vi "Three part faster sub note on off.vi"() -> ()   [LabVIEW 2009]
uses:
  <vilib>/vision/Image Controls.llb/IMAQ Image.ctl
  <vilib>/Instr/_visa.llb/VISA Configure Serial Port (Instr).vi
  <vilib>/vision/NI_Vision_Development_Module.lvlib
panel:
  in  "Notes On/OFF":bool
  in  "VISA resource name":refnum<visa-resource-name>
  out "number":u8 format="%b"
  out "decimal integer string":string
  out "decimal integer string 2":string
  out "decimal integer string 3":string
  out "number 2":u8 format="%b"
  out "number 3":u8 format="%b"
  out "Guitar Cluster":T1
  out "Bass Cluster":T2
  out "Drum Cluster":T3
  out "Image 2":T4(plugin-control)
  in  "Orange Bass":T5={"Global Rectangle"=[220, 302, 227, 392], "Contours"=[{"ID"=enum."External", "Type"=2, "Coordinates"=[226, 391, 220, 302]}]} {"Contours"."Type" items=["No Selection", "Point", "Line", "Rectangle", "Oval", "Polygon", "Freehand Region", "Annulus", "Unused2", "Unused3", "Broken Line", "Freehand Line", "Rotated Rectangle"]}
  in  "Blue Bass":T5={"Global Rectangle"=[192, 292, 199, 386], "Contours"=[{"ID"=enum."External", "Type"=2, "Coordinates"=[192, 385, 198, 292]}]} {"Contours"."Type" items=["No Selection", "Point", "Line", "Rectangle", "Oval", "Polygon", "Freehand Region", "Annulus", "Unused2", "Unused3", "Broken Line", "Freehand Line", "Rotated Rectangle"]}
  in  "playtime":dbl=30.0
  in  "Orange Guitar":T5={"Global Rectangle"=[587, 282, 628, 378], "Contours"=[{"ID"=enum."External", "Type"=2, "Coordinates"=[627, 377, 587, 282]}]} {"Contours"."Type" items=["No Selection", "Point", "Line", "Rectangle", "Oval", "Polygon", "Freehand Region", "Annulus", "Unused2", "Unused3", "Broken Line", "Freehand Line", "Rotated Rectangle"]}
  in  "Yellow Guitar":T5={"Global Rectangle"=[546, 282, 563, 376], "Contours"=[{"ID"=enum."External", "Type"=2, "Coordinates"=[562, 375, 546, 282]}]} {"Contours"."Type" items=["No Selection", "Point", "Line", "Rectangle", "Oval", "Polygon", "Freehand Region", "Annulus", "Unused2", "Unused3", "Broken Line", "Freehand Line", "Rotated Rectangle"]}
  in  "Green Guitar":T5={"Global Rectangle"=[498, 284, 505, 376], "Contours"=[{"ID"=enum."External", "Type"=2, "Coordinates"=[498, 375, 504, 284]}]} {"Contours"."Type" items=["No Selection", "Point", "Line", "Rectangle", "Oval", "Polygon", "Freehand Region", "Annulus", "Unused2", "Unused3", "Broken Line", "Freehand Line", "Rotated Rectangle"]}
  in  "Blue Guitar":T5={"Global Rectangle"=[569, 290, 594, 372], "Contours"=[{"ID"=enum."External", "Type"=2, "Coordinates"=[593, 371, 569, 290]}]} {"Contours"."Type" items=["No Selection", "Point", "Line", "Rectangle", "Oval", "Polygon", "Freehand Region", "Annulus", "Unused2", "Unused3", "Broken Line", "Freehand Line", "Rotated Rectangle"]}
  in  "Red Guitar":T5={"Global Rectangle"=[526, 284, 530, 370], "Contours"=[{"ID"=enum."External", "Type"=2, "Coordinates"=[529, 369, 526, 284]}]} {"Contours"."Type" items=["No Selection", "Point", "Line", "Rectangle", "Oval", "Polygon", "Freehand Region", "Annulus", "Unused2", "Unused3", "Broken Line", "Freehand Line", "Rotated Rectangle"]}
  in  "Green Bass":T5={"Global Rectangle"=[100, 292, 131, 371], "Contours"=[{"ID"=enum."External", "Type"=2, "Coordinates"=[100, 370, 130, 292]}]} {"Contours"."Type" items=["No Selection", "Point", "Line", "Rectangle", "Oval", "Polygon", "Freehand Region", "Annulus", "Unused2", "Unused3", "Broken Line", "Freehand Line", "Rotated Rectangle"]}
  in  "Red Bass":T5={"Global Rectangle"=[129, 294, 154, 376], "Contours"=[{"ID"=enum."External", "Type"=2, "Coordinates"=[129, 375, 153, 294]}]} {"Contours"."Type" items=["No Selection", "Point", "Line", "Rectangle", "Oval", "Polygon", "Freehand Region", "Annulus", "Unused2", "Unused3", "Broken Line", "Freehand Line", "Rotated Rectangle"]}
  in  "Yellow Bass":T5={"Global Rectangle"=[160, 295, 175, 378], "Contours"=[{"ID"=enum."External", "Type"=2, "Coordinates"=[160, 377, 174, 295]}]} {"Contours"."Type" items=["No Selection", "Point", "Line", "Rectangle", "Oval", "Polygon", "Freehand Region", "Annulus", "Unused2", "Unused3", "Broken Line", "Freehand Line", "Rotated Rectangle"]}
  out "Image Dst Out":T4
  out "Frame Number":i32
  in  "Frame Start":i32
  in  "stop":bool
  in  "AVI Path":path
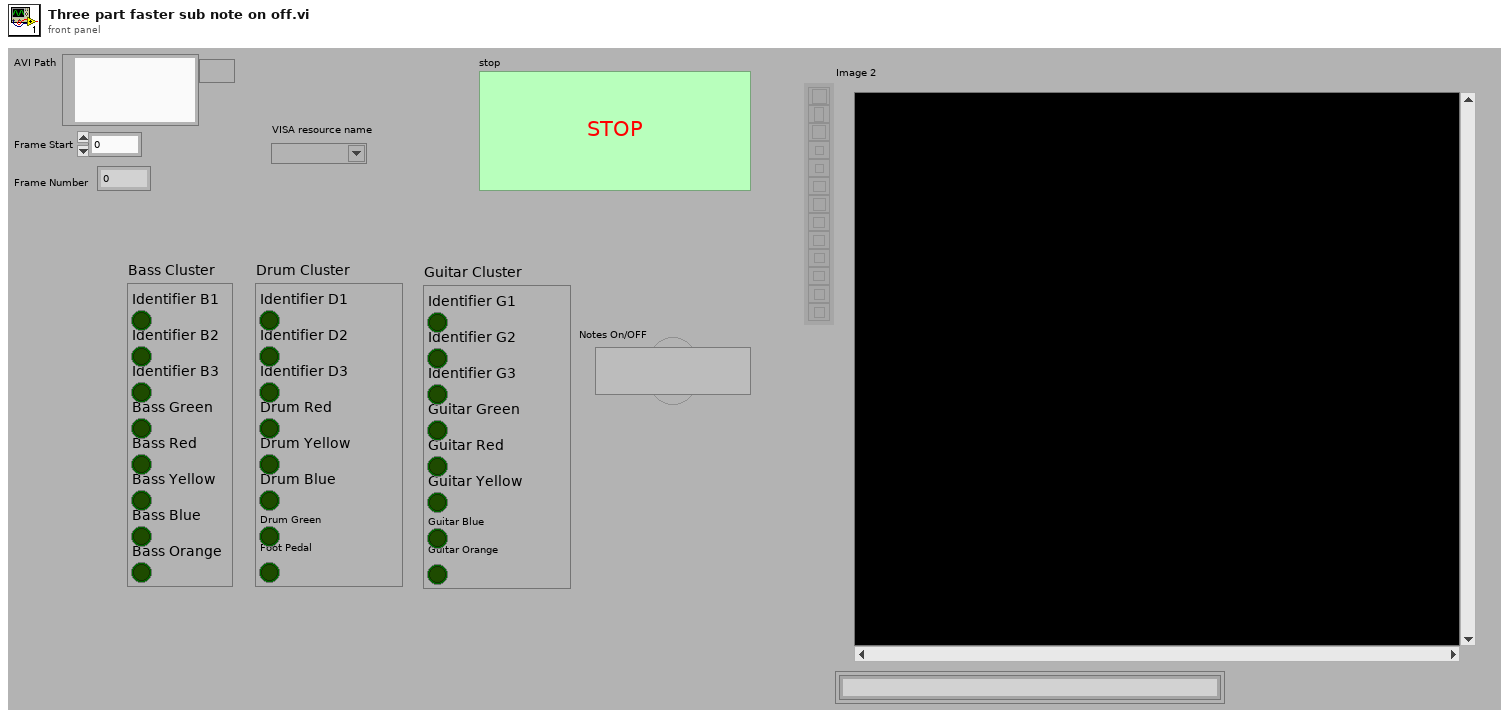
[diagram p1: front panel]
types:
  T1 = cluster{"Identifier G1":bool, "Identifier G2":bool, "Identifier G3":bool, "Guitar Green":bool, "Guitar Red":bool, "Guitar Yellow":bool, "Guitar Blue":bool, "Guitar Orange":bool}
  T2 = cluster{"Identifier B1":bool, "Identifier B2":bool, "Identifier B3":bool, "Bass Green":bool, "Bass Red":bool, "Bass Yellow":bool, "Bass Blue ":bool, "Bass Orange":bool}
  T3 = cluster{"Identifier D1":bool, "Identifier D2":bool, "Identifier D3":bool, "Drum Red":bool, "Drum Yellow":bool, "Drum Blue":bool, "Drum Green":bool, "Foot Pedal":bool}
  T4 = typedef "IMAQ Image.ctl" = refnum<image>
  T5 = cluster{"Global Rectangle":i32[], "Contours":cluster{"ID":enum32{"External", "Internal"}, "Type":u32, "Coordinates":i32[]}[]}
  T6 = typedef "Image Type" = u32
  T7 = typedef "AviRefnum.ctl" = refnum<k1>
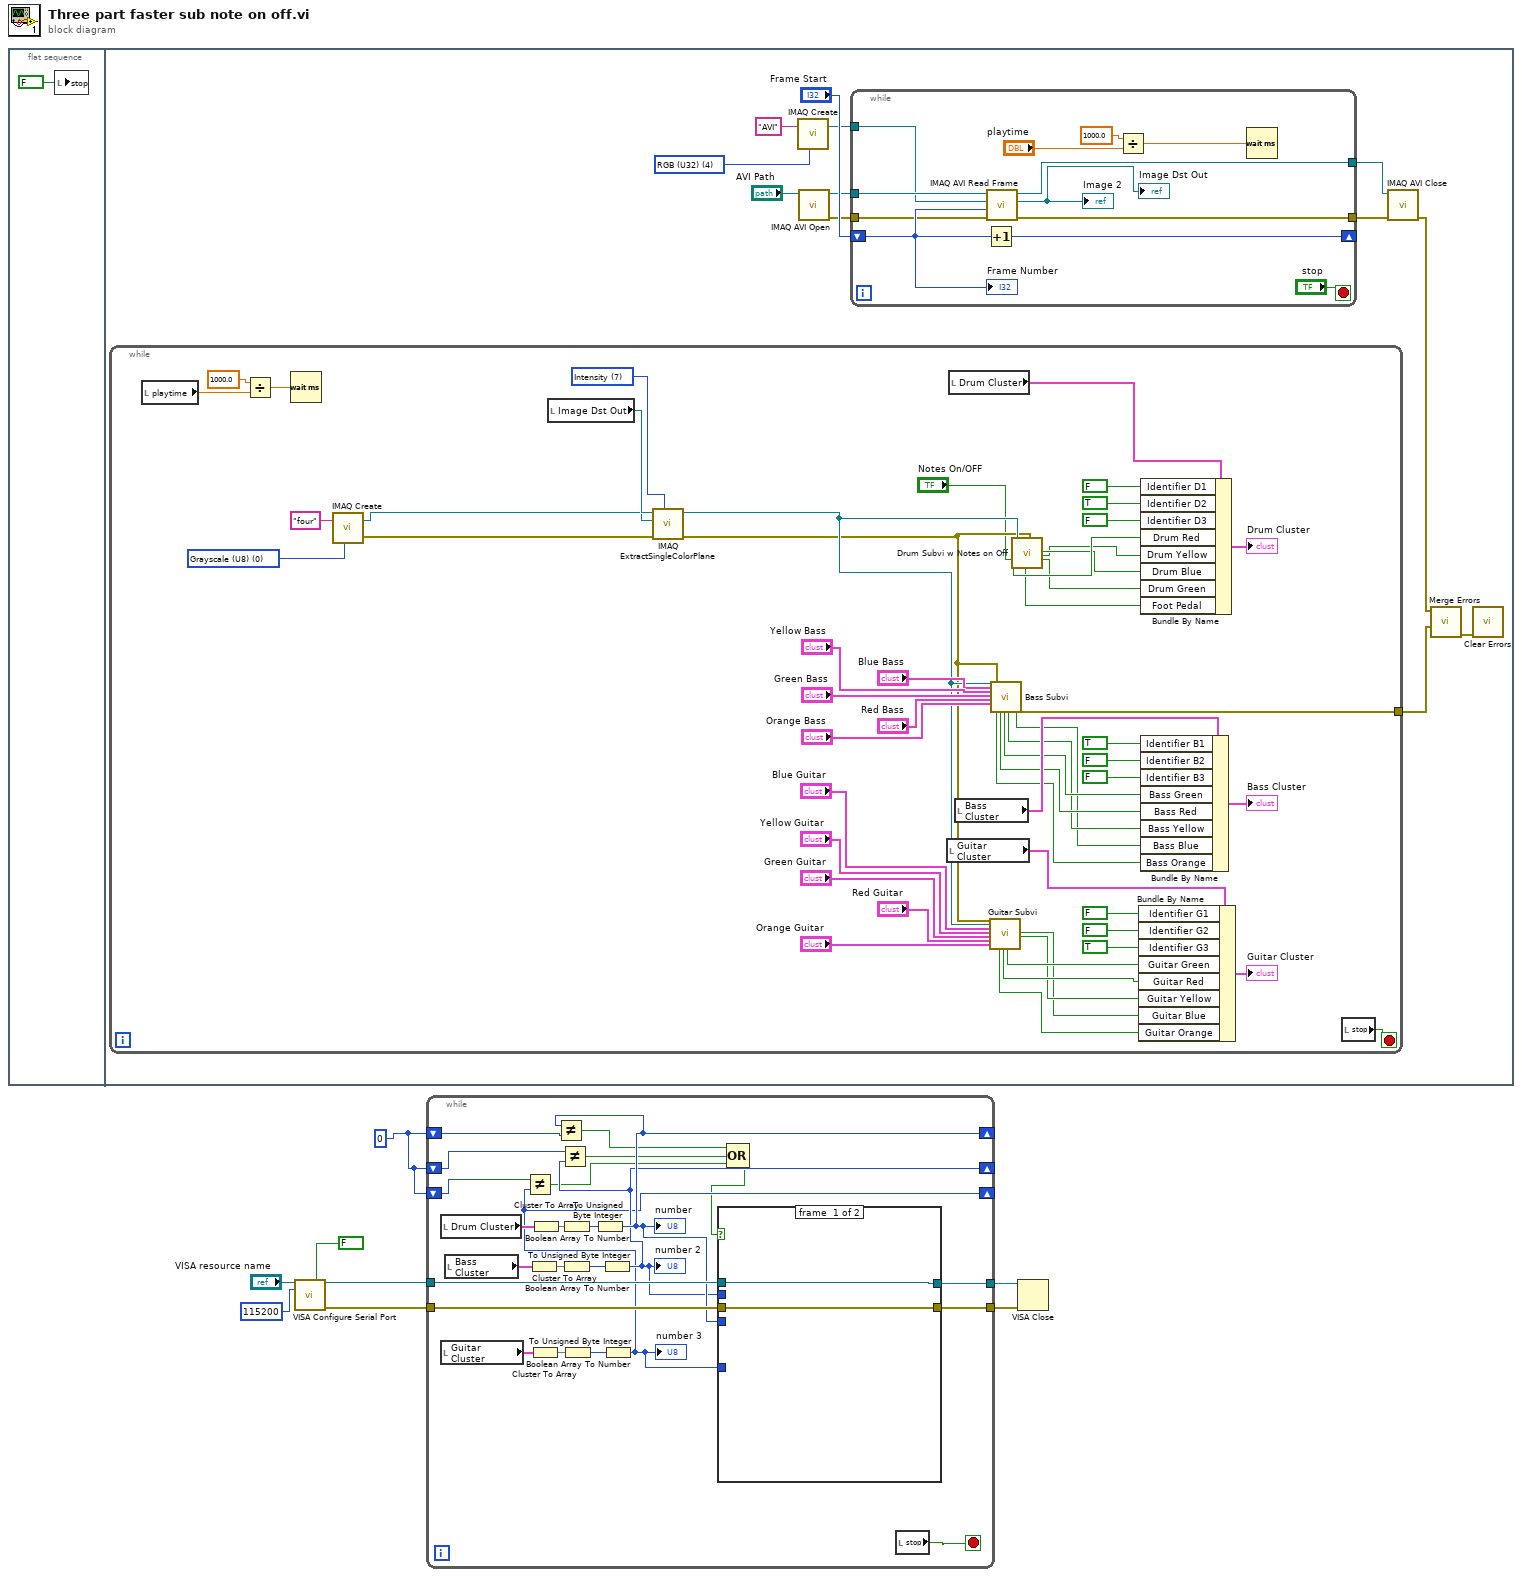
[diagram p0: block diagram]
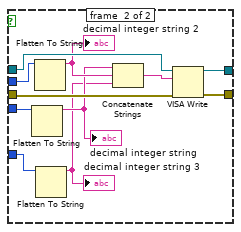
[diagram p2: hidden frame]
diagram:
  w1 = u8 0
  n1 = flat-sequence {
    frame #0 {
      n2 = local write "stop"(FALSE ("stop")) -> ()
    }
    frame #1 {
      w13 = T6 4 items=["Grayscale (U8)", "Grayscale (I16)", "Grayscale (SGL)", "Complex (CSG)", "RGB (U32)", "HSL (U32)", "RGB (U64)", "Grayscale (U16)"] ("Image Type")
      n3 = while {
        tunnel: [w65] -> w10
        stop <- w74 stop-if-true
        w70 = T6 0 items=["Grayscale (U8)", "Grayscale (I16)", "Grayscale (SGL)", "Complex (CSG)", "RGB (U32)", "HSL (U32)", "RGB (U64)", "Grayscale (U16)"] ("Image Type")
        w75 = 7 items=["Red", "Green", "Blue", "Hue", "Saturation", "Luminance", "Value", "Intensity"] ("Color Plane")
        n4 = local read "playtime"() -> (w59:dbl)
        n5 = Divide(x=1000.0, y=w59) -> (x/y=w73:dbl)
        n6 = Wait (ms)(milliseconds to wait=w73) -> ()  [unwired: 1 out]
        n7 = call "IMAQ Create"("Image Name"="four", "Image Type"=w70) -> ("New Image"=w31:T4, "error out"=w30:errorcluster)  [unwired: 3 in]
        n8 = local read "Image Dst Out"() -> (w71:T4)
        n9 = call "IMAQ ExtractSingleColorPlane"("Color Plane"=w75, "error in (no error)"=w30, "Image Dst"=w31, "Image Src"=w71) -> ("error out"=w26:errorcluster, "Image Dst Out"=w29:T4)  [unwired: 6 out]
        n10 = local read "Guitar Cluster"() -> (w40:T1)
        n11 = local read "Drum Cluster"() -> (w55:T3)
        n12 = local read "Bass Cluster"() -> (w51:T2)
        n13 = call "Guitar Subvi.vi"("error out"=w26, "Image Dst Out"=w29, "Blue Guitar 2"="Blue Guitar", "Yellow Guitar 2"="Yellow Guitar", "Green Guitar 2"="Green Guitar", "Red Guitar 2"="Red Guitar", "Orange Guitar 2"="Orange Guitar") -> ("Orange Guitar LED"=w32:bool, "Red Guitar LED"=w35:bool, "Green Guitar LED"=w36:bool, "Blue Guitar LED"=w33:bool, "Yellow Guitar LED"=w34:bool)  [unwired: 16 in]
        n14 = call "Bass Subvi.vi"("Image Dst Out"=w29, "Blue Bass 2"="Blue Bass", "Yellow Bass 2"="Yellow Bass", "Green Bass 2"="Green Bass", "Red Bass 2"="Red Bass", "Orange Bass 2"="Orange Bass", "error out"=w26) -> ("Orange Bass LED"=w42:bool, "Red Bass LED"=w45:bool, "Green Bass LED"=w46:bool, "Yellow Bass LED"=w44:bool, "Blue Bass LED"=w43:bool, "error out 2"=w65:errorcluster)  [unwired: 15 in]
        n15 = call "Drum Subvi w Notes on Off.vi"("Drum Notes On/Off"="Notes On/OFF", "Image Dst Out"=w29, "error out"=w26) -> ("Red Drum"=w28:bool, "Foot Pedal"=w27:bool, "Blue Drum 2"=w25:bool, "Yellow Drum"=w23:bool, "Green Drum"=w24:bool)  [unwired: 15 in, 5 out]
        n16 = Bundle By Name(cluster=w40, "Identifier G1"=FALSE ("element"), "Identifier G2"=FALSE ("element"), "Identifier G3"=TRUE ("element"), "Guitar Green"=w36, "Guitar Red"=w35, "Guitar Yellow"=w34, "Guitar Blue"=w33, "Guitar Orange"=w32) -> (→"Guitar Cluster":T1)
        n17 = Bundle By Name(cluster=w55, "Identifier D1"=FALSE ("D1"), "Identifier D2"=TRUE ("D2"), "Identifier D3"=FALSE ("D3"), "Drum Red"=w28, "Drum Yellow"=w23, "Drum Blue"=w25, "Drum Green"=w24, "Foot Pedal"=w27) -> (→"Drum Cluster":T3)
        n18 = Bundle By Name(cluster=w51, "Identifier B1"=TRUE, "Identifier B2"=FALSE ("element"), "Identifier B3"=FALSE ("element"), "Bass Green"=w46, "Bass Red"=w45, "Bass Yellow"=w44, "Bass Blue"=w43, "Bass Orange"=w42) -> (→"Bass Cluster":T2)
        n19 = local read "stop"() -> (w74:bool)
      }
      n20 = call "IMAQ Create"("Image Name"="AVI", "Image Type"=w13) -> ("New Image"=w11:T4)  [unwired: 3 in, 1 out]
      n21 = call "IMAQ AVI Open"("AVI Path"="AVI Path") -> ("error out"=w18:errorcluster, "Avi Refnum"=w19:T7)  [unwired: 9 in]
      n22 = while {
        tunnel: w19 -> [w87]
        tunnel: w18 -> [w79]
        tunnel: [w86] -> w20
        shift-right: [w81] -> _
        shift-left: "Frame Start" -> [w80]
        tunnel: [w78] -> w14
        tunnel: w11 -> [w77]
        stop <- "stop" stop-if-true
        n23 = Increment(x=w80) -> (x+1=w81:i32)
        n24 = call "IMAQ AVI Read Frame"("error in (no error)"=w79, "Frame Number"=w80, "Image"=w77, "Avi Refnum"=w87) -> ("error out"=w78:errorcluster, "Image Out"=→"Image Dst Out" →"Image 2":T4, "Avi Refnum (duplicate)"=w86:T7)  [unwired: 4 in, 1 out]
        n25 = Divide(x=1000.0, y="playtime") -> (x/y=w84:dbl)
        n26 = Wait (ms)(milliseconds to wait=w84) -> ()  [unwired: 1 out]
        "Frame Number" <- w80
      }
      n27 = call "IMAQ AVI Close"("error in (no error)"=w14, "Avi Refnum"=w20) -> ("error out"=w16:errorcluster)  [unwired: 9 in]
      n28 = call <vilib>:"Merge Errors.vi"("error in 3 (no error)"=w10, "error in 1 (no error)"=w16) -> ("error out"=w15:errorcluster)  [unwired: 5 in]
      n29 = call <vilib>:"Clear Errors.vi"("error in (no error)"=w15) -> ()  [unwired: 6 in, 1 out]
    }
  }
  n30 = call-poly "VISA Configure Serial Port"("VISA resource name"="VISA resource name", "Enable Termination\nChar (T)"=FALSE ("Enable Termination\nChar (T)"), "baud rate (9600)"=u32 115200) -> ("VISA resource name out"=w8:refnum<visa-resource-name>, "error out"=w3:errorcluster)  [unwired: 11 in]
  n31 = while {
    tunnel: w8 -> [w111]
    tunnel: [w110] -> w7
    tunnel: w3 -> [w109]
    tunnel: [w108] -> w2
    shift-right: [w100] -> _
    shift-left: w1 -> [w99]
    shift-right: [w98] -> _
    shift-left: w1 -> [w97]
    shift-right: [w92] -> _
    shift-left: w1 -> [w93]
    stop <- w103 stop-if-true
    n32 = local read "Drum Cluster"() -> (w104:T3)
    n33 = local read "Guitar Cluster"() -> (w95:T1)
    n34 = local read "Bass Cluster"() -> (w105:T2)
    n35 = Cluster To Array(cluster=w105) -> (array=w106:bool[])
    n36 = Cluster To Array(cluster=w95) -> (array=w94:bool[])
    n37 = Cluster To Array(cluster=w104) -> (array=w107:bool[])
    n38 = Boolean Array To Number(Boolean array=w107) -> (number=w102:u32)
    n39 = Boolean Array To Number(Boolean array=w106) -> (number=w101:u32)
    n40 = Boolean Array To Number(Boolean array=w94) -> (number=w96:u32)
    n41 = To Unsigned Byte Integer(number=w102) -> (unsigned 8bit integer=w100:u8)
    "number" <- w100
    n42 = Not Equal?(x=w100, y=w99) -> (x != y?=w90:bool)
    n43 = To Unsigned Byte Integer(number=w101) -> (unsigned 8bit integer=w98:u8)
    "number 2" <- w98
    n44 = Not Equal?(x=w97, y=w98) -> (x != y?=w89:bool)
    n45 = To Unsigned Byte Integer(number=w96) -> (unsigned 8bit integer=w92:u8)
    "number 3" <- w92
    n46 = Not Equal?(x=w93, y=w92) -> (x != y?=w88:bool)
    n47 = Compound Arithmetic op=OR(w90, w89, w88) -> (w91:bool)
    n48 = case shown="True" w91 {
      tunnel: w111 -> [w113 w124]
      tunnel: [w113 w123] -> w110
      tunnel: w100 -> [_ w117]
      tunnel: w109 -> [w112 w122]
      tunnel: [w112 w121] -> w108
      tunnel: w98 -> [_ w119]
      tunnel: w92 -> [_ w114]
      frame #0 {
      }
      frame #1 {
        n49 = Flatten To String(anything=w117) -> (data string=w116:string)  [unwired: 3 in, 2 out]
        "decimal integer string" <- w116
        n50 = Flatten To String(anything=w119) -> (data string=w118:string)  [unwired: 3 in, 2 out]
        "decimal integer string 2" <- w118
        n51 = Flatten To String(anything=w114) -> (data string=w115:string)  [unwired: 3 in, 2 out]
        "decimal integer string 3" <- w115
        n52 = Concatenate Strings(w116, w118, w115) -> (w120:string)
        n53 = VISA Write(VISA resource name=w124, write buffer=w120, error in (no error)=w122) -> (VISA resource name out=w123:refnum<visa-resource-name>, error out=w121:errorcluster)  [unwired: 1 out]
      }
    }
    n54 = local read "stop"() -> (w103:bool)
  }
  n55 = VISA Close(VISA resource name=w7, error in (no error)=w2) -> ()  [unwired: 1 out]
